vi "FittedCurvePolynom.vi"() -> ()   [LabVIEW 2012]
panel:
  in  "FittedCurvePolynom":dbl[](array[numeric])
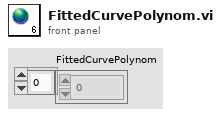
[diagram p1: front panel]
diagram:
